vi "Test State.vi"(8 "error in (no error)":errorcluster, 10 "Assert Event Data":T1={"name"="", "passed"=FALSE, "call-chain"=[], "test-error"={"status"=FALSE, "code"=0, "source"=""}, "timestamp"=timestamp(0 s since 1904-01-01), "assert-id"="", "test-id"="", "time"=-1.0, "message"="", "properties"=variant, "measurements"=variant, "user-defined"=variant}) -> (0 "error out":errorcluster, 3 "Test State":T2)   [LabVIEW 2013, in "Caraya.lvlib" / "Basic Test Manager.lvclass"]
uses:
  Basic Test Manager.lvclass
  Test State.ctl
  Test Result/Assert Event Data (Extended).ctl
  Test Result/Test Result.lvclass
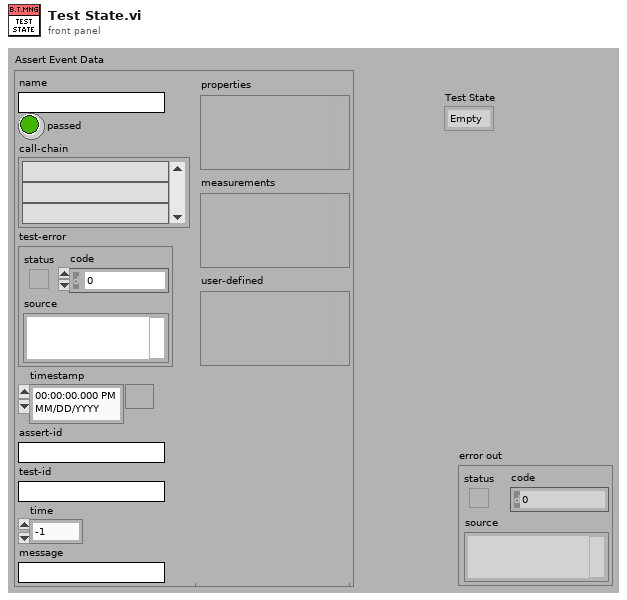
[diagram p1: front panel]
types:
  T1 = typedef "Caraya.lvlib/Test Result.lvclass/Assert Event Data (Extended).ctl" = cluster{"name":string, "passed":bool, "call-chain":string[], "test-error":errorcluster, "timestamp":timestamp, "assert-id":string, "test-id":string, "time":dbl, "message":string, "properties":variant, "measurements":variant, "user-defined":variant}
  T2 = typedef "Caraya.lvlib/Basic Test Manager.lvclass/Test State.ctl" = enum16{"Empty", "Unknown", "Fail", "Pass", "Skip", "Error"}
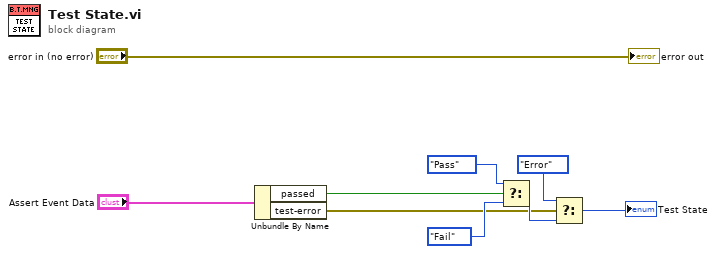
[diagram p0: block diagram]
diagram:
  n1 = Unbundle By Name("Assert Event Data") -> ("passed"=w3:bool, "test-error"=w2:errorcluster)
  n2 = Select(t=Test_State."Pass" ("Enum"), s=w3, f=Test_State."Fail" ("Enum")) -> (s? t:f=w8:T2)
  n3 = Select(t=Test_State."Error" ("Enum"), s=w2, f=w8) -> (s? t:f=→"Test State":T2)
  "error out" <- "error in (no error)"
